vi "电压读取设备选取.vi"(8 "error out":errorcluster, 10 "布尔":bool, 11 "电压读取":refnum<visa-resource-name>) -> (0 "error out 2":errorcluster caption="error out", 2 "所有匹配":string, 3 "VISA resource name out":refnum<visa-resource-name>)   [LabVIEW 2021]
uses:
  <vilib>/regexp/Match Regular Expression.xnode
  <instrlib>/Keithley DMM6500 DAQ6500 Series/Keithley DMM6500 DAQ6500 Series.lvlib
  <instrlib>/Keithley DMM7510/Keithley DMM7510.lvlib
  <instrlib>/Keithley 27XX/Keithley 27XX.lvlib
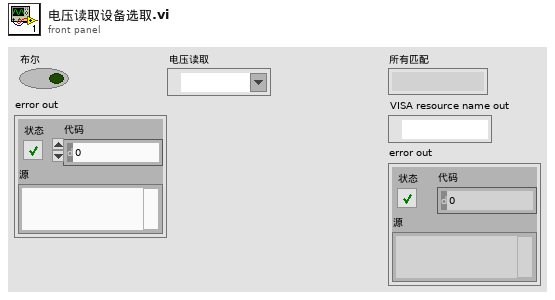
[diagram p1: front panel]
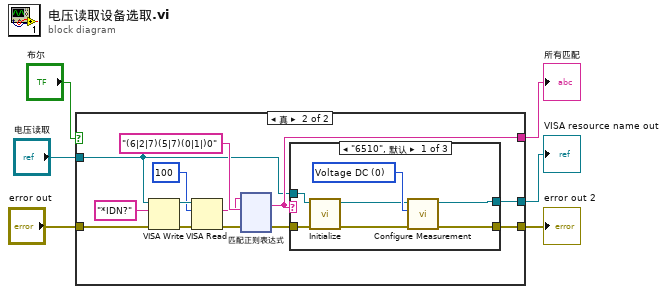
[diagram p0: block diagram]
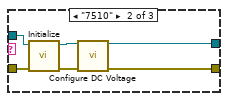
[diagram p3: hidden frame]
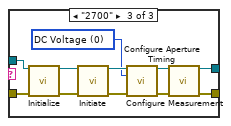
[diagram p4: hidden frame]
diagram:
  n1 = case shown="真" "布尔" {
    tunnel: "error out" -> [w7 w12]
    tunnel: [w7 w11] -> w1
    tunnel: [_ w10] -> w3
    tunnel: [_ w9] -> w2
    tunnel: "电压读取" -> [_ w8]
    frame False {
    }
    frame True {
      n2 = VISA Write(VISA resource name=w8, write buffer="*IDN?" ("写入缓冲区"), error in (no error)=w12) -> (VISA resource name out=w18:refnum<visa-resource-name>, error out=w19:errorcluster)  [unwired: 1 out]
      n3 = VISA Read(VISA resource name=w18, byte count=u32 100 ("字节总数"), error in (no error)=w19) -> (read buffer=w15:string, error out=w14:errorcluster)  [unwired: 2 out]
      n4 = xnode "匹配正则表达式"("输入字符串"=w15, "正则表达式"="(6|2|7)(5|7)(0|1|)0", "错误输入"=w14) -> ("所有匹配"=w10:string, "错误输出"=w13:errorcluster)  [unwired: 3 in, 3 out]
      n5 = case shown="\"6510\", 默认" w10 {
        tunnel: w8 -> [w143 w150 w161]
        tunnel: w13 -> [w140 w145 w156]
        tunnel: [w139 w147 w155] -> w9
        tunnel: [w138 w146 w153] -> w11
        frame "6510", Default {
          w144 = 0 items=["Voltage DC", "Voltage AC", "Current DC", "Current AC", "Resistance", "4-wire Resistance", "Diode", "Capacitance", "Temperature", "Continuity", "Frequency", "Period", "Voltage Ratio", "Voltage", "Current"] ("Function (0: Voltage DC)")
          n6 = call <instrlib>:"Initialize.vi"("error in (no error)"=w140, "VISA resource name"=w143) -> ("error out"=w141:errorcluster, "VISA resource name out"=w142:refnum<visa-resource-name>)  [unwired: 8 in]
          n7 = call <instrlib>:"Configure Measurement.vi"("error in (no error)"=w141, "Function (0: Voltage DC)"=w144, "VISA resource name"=w142) -> ("error out"=w138:errorcluster, "VISA resource name out"=w139:refnum<visa-resource-name>)  [unwired: 7 in]
        }
        frame "7510" {
          n8 = call <instrlib>:"Initialize.vi"("error in (no error)"=w145, "VISA resource name"=w150) -> ("error out"=w148:errorcluster, "VISA resource name out"=w149:refnum<visa-resource-name>)  [unwired: 8 in]
          n9 = call <instrlib>:"Configure DC Voltage.vi"("VISA resource name"=w149, "error in (no error)"=w148) -> ("VISA resource name out"=w147:refnum<visa-resource-name>, "error out"=w146:errorcluster)  [unwired: 12 in]
        }
        frame "2700" {
          w157 = u16 0 items=["DC Voltage", "AC Voltage", "DC Current", "AC Current", "Resistance", "Four-Wire Resistance", "Temperature", "Frequency", "Period", "Continuity"] ("Function (0: DC Voltage)")
          n10 = call <instrlib>:"Initialize.vi"("VISA resource name"=w161, "error in (no error)"=w156) -> ("VISA resource name out"=w160:refnum<visa-resource-name>, "error out"=w152:errorcluster)  [unwired: 12 in]
          n11 = call <instrlib>:"Initiate.vi"("VISA resource name"=w160, "error in (no error)"=w152) -> ("VISA resource name out"=w159:refnum<visa-resource-name>, "error out"=w151:errorcluster)  [unwired: 12 in]
          n12 = call <instrlib>:"Configure Measurement.vi"("VISA resource name"=w159, "Function (0: DC Voltage)"=w157, "error in (no error)"=w151) -> ("VISA resource name out"=w158:refnum<visa-resource-name>, "error out"=w154:errorcluster)  [unwired: 11 in]
          n13 = call <instrlib>:"Configure Aperture Timing.vi"("VISA resource name"=w158, "error in (no error)"=w154) -> ("VISA resource name out"=w155:refnum<visa-resource-name>, "error out"=w153:errorcluster)  [unwired: 12 in]
        }
      }
    }
  }
  "所有匹配" <- w3
  "VISA resource name out" <- w2
  "error out 2" <- w1
